vi "Reserve Session(s).vi"   [LabVIEW 2020, in "NIDCPowerSourceDCVoltage.lvlib"]
uses:
  NIDCPowerSourceDCVoltage.lvlib
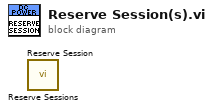
[diagram p0: block diagram]
diagram:
  n1 = call "Reserve Sessions.vi"() -> ()  [unwired: 7 in, 5 out]
  n2 = call "Reserve Session.vi"() -> ()  [unwired: 7 in, 5 out]
